vi "Write Path.vi"(8 "error in (no error)":errorcluster, 9 "File (Configuration.ini)":string="Configuration.ini", 10 "Path":path, 11 "Configuration in":refnum<class "Configuration.lvclass">) -> (0 "error out":errorcluster, 3 "Configuration out":refnum<class "Configuration.lvclass">)   [LabVIEW 2016, in "Configuration.lvclass"]
uses:
  Configuration.lvclass
  Configuration.lvclass/Configuration.ctl
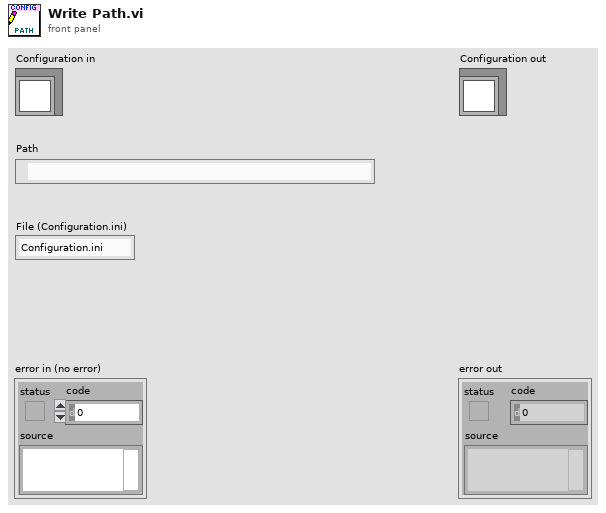
[diagram p1: front panel]
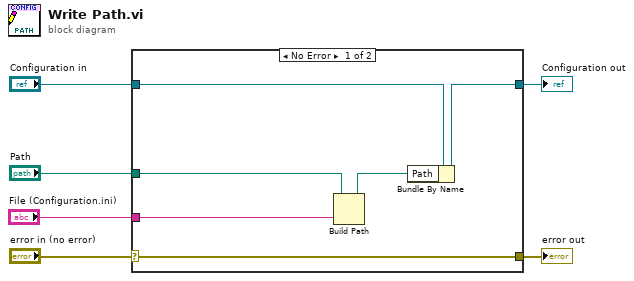
[diagram p0: block diagram]
diagram:
  n1 = case shown="No Error" "error in (no error)" {
    selector: "error in (no error)" -> [w12 w13]
    tunnel: [w12 w13] -> w5
    tunnel: [w10 w14] -> w3
    tunnel: "Configuration in" -> [w11 w14]
    tunnel: "Path" -> [w9 _]
    tunnel: "File (Configuration.ini)" -> [w7 _]
    frame No Error {
      n2 = Build Path(base path=w9, name or relative path=w7) -> (appended path=w8:path)
      n3 = Bundle By Name(cluster=w11, "Path"=w8) -> (w10:refnum<class "Configuration.lvclass">)
    }
    frame Error {
    }
  }
  "error out" <- w5
  "Configuration out" <- w3
